vi "Trigger.vi"() -> ()   [LabVIEW 2014]
panel:
  in  "ICImagingControl":refnum<k7>(container)
  out "Picture Out":picture
  in  "Open Device Configuration (Monochrome  Images)":bool
  in  "Open Device Configuration (Color Images)":bool
  out "ReferenceTimeStart":dbl
  out "Image Age":dbl
  out "ReferenceTimeCurrent":dbl
  out "SampleStartTime":dbl
  in  "External Trigger":bool
  in  "Grab":bool
  in  "End Program":bool
  # "Open Device Configuration"
  # "Off"
  # "On"
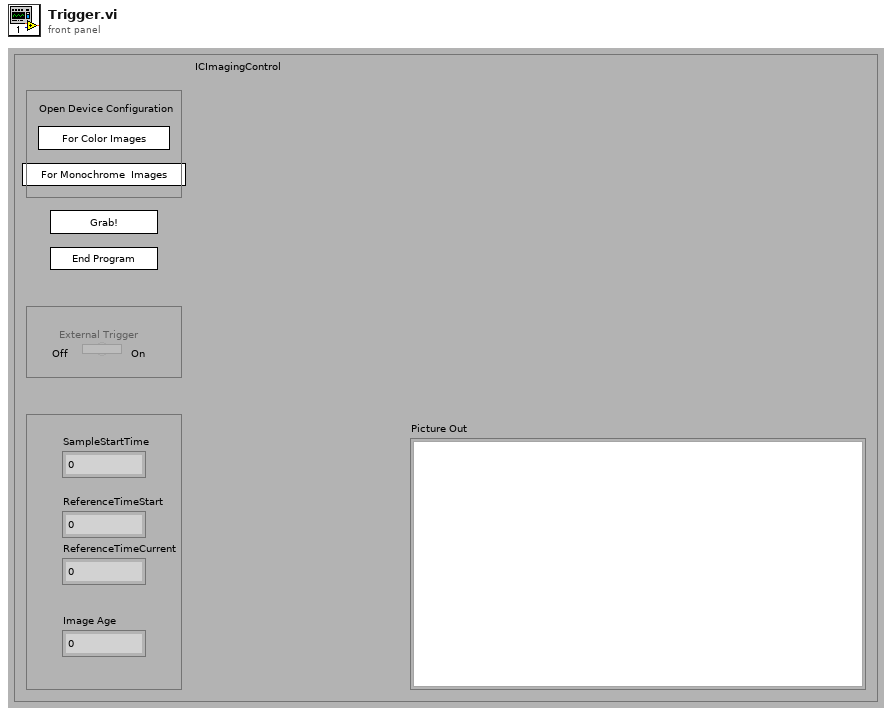
[diagram p1: front panel]
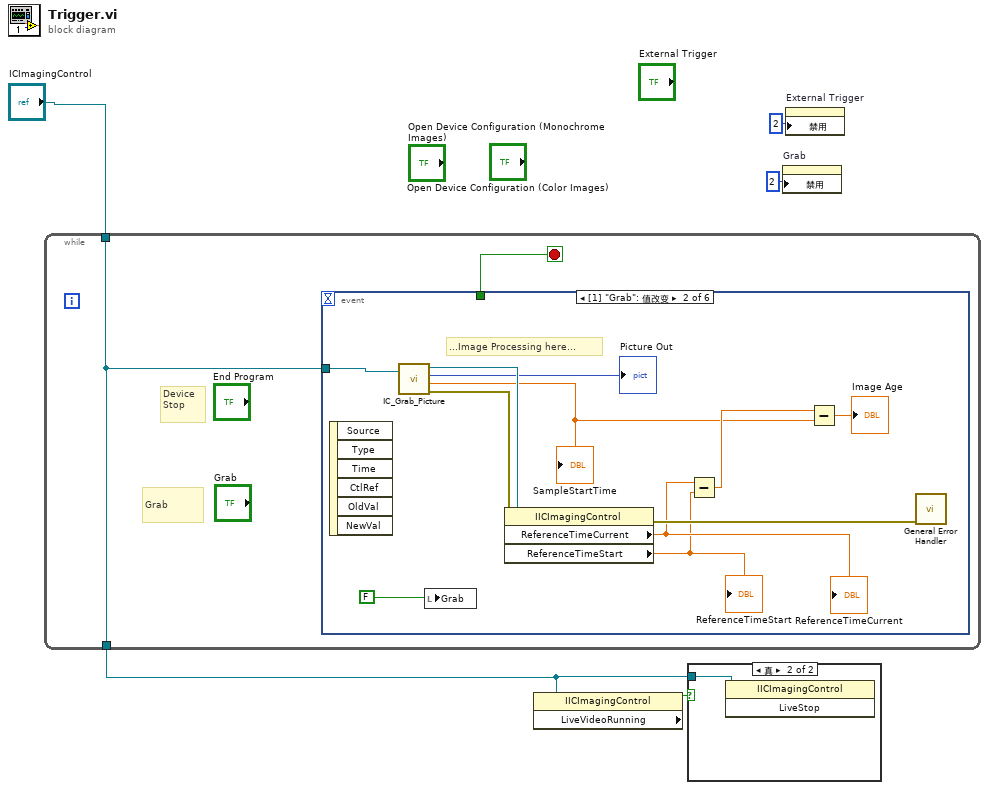
[diagram p0: block diagram]
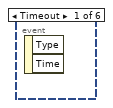
[diagram p3: hidden frame]
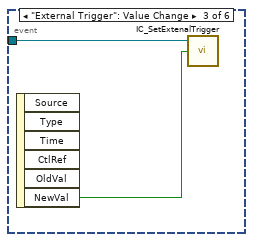
[diagram p4: hidden frame]
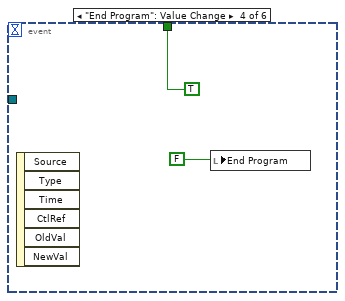
[diagram p5: hidden frame]
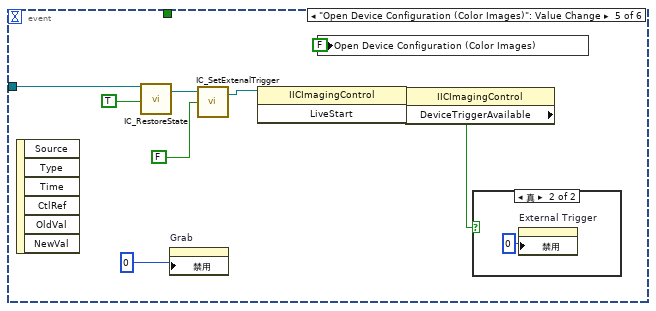
[diagram p6: hidden frame]
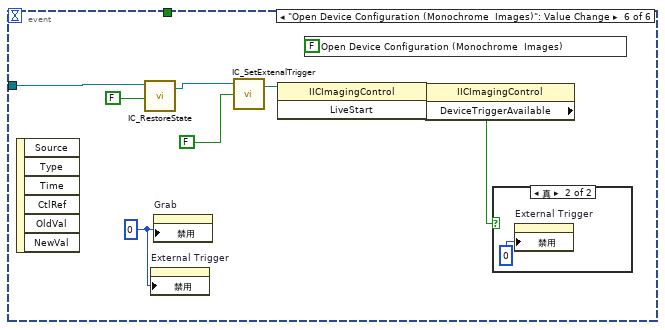
[diagram p8: hidden frame]
diagram:
  n1 = while {
    tunnel: "ICImagingControl" -> [w6]
    tunnel: [w6] -> w4
    stop <- w7 stop-if-true
    # "Device\nStop"
    # "Grab"
    n2 = event shown="[1] \"Grab\": 值改变" {
      selector: _ -> [_ _ _ _ _ _]
      dyn-events: _ -> [_ _ _ _ _ _]
      timeout: _ -> [_ _ _ _ _ _]
      tunnel: w6 -> [_ w17 w20 _ w31 w40]
      tunnel: [_ _ _ TRUE _ _] -> w7
      event Timeout {
        n3 = event-data() -> ()  [unwired: 1 in, 2 out]
      }
      event "Grab": Value Change {
        # "...Image Processing here..."
        n4 = event-data() -> ()  [unwired: 1 in, 6 out]
        n5 = call "IC_Grab_Picture.vi"("ICImagingControl In"=w17) -> ("ICImagingControl Out"=w16:refnum<k7>, "Picture Out"=→"Picture Out":picture, "SampleStartTime"=w11:dbl, "Error Out"=w13:errorcluster)  [unwired: 1 in]
        "SampleStartTime" <- w11
        n6 = local write "Grab"(FALSE) -> ()
        n7 = property class="IICImagingControl"(reference=w16, error in=w13) -> (error out=w14:errorcluster, "ReferenceTimeCurrent"=w10:dbl, "ReferenceTimeStart"=w9:dbl)  [unwired: 1 out]
        "ReferenceTimeCurrent" <- w10
        "ReferenceTimeStart" <- w9
        n8 = Subtract(x=w10, y=w9) -> (x-y=w12:dbl)
        n9 = Subtract(x=w12, y=w11) -> (x-y=→"Image Age":dbl)
        n10 = call <vilib>:"General Error Handler.vi"("error in (no error)"=w14) -> ()  [unwired: 10 in, 5 out]
      }
      event "External Trigger": Value Change {
        n11 = event-data() -> ("NewVal"=w19:bool)  [unwired: 1 in, 5 out]
        n12 = call <userlib>:"IC_SetExtenalTrigger.vi"("Trigger"=w19, "ICImagingControl In"=w20) -> ()  [unwired: 1 in, 2 out]
      }
      event "End Program": Value Change {
        n13 = event-data() -> ()  [unwired: 1 in, 6 out]
        n14 = local write "End Program"(FALSE) -> ()
      }
      event "Open Device Configuration (Color Images)": Value Change {
        n15 = event-data() -> ()  [unwired: 1 in, 6 out]
        n16 = call "IC_RestoreState.vi"("Color"=TRUE, "ICImagingControl"=w31) -> ("ICImagingControl Out"=w23:refnum<k7>)  [unwired: 2 in, 1 out]
        n17 = property on="Grab" class="Bool (严格)"("禁用"=0) -> ()  [unwired: 2 in, 2 out]
        n18 = call <userlib>:"IC_SetExtenalTrigger.vi"("Trigger"=FALSE, "ICImagingControl In"=w23) -> ("ICImagingControl Out"=w24:refnum<k7>)  [unwired: 1 in, 1 out]
        n19 = invoke class="IICImagingControl" method="LiveStart"(reference=w24) -> (reference out=w26:refnum<k7>)  [unwired: 2 in, 2 out]
        n20 = local write "Open Device Configuration (Color Images)"(FALSE ("Open Device Configuration (Color Images)")) -> ()
        n21 = property class="IICImagingControl"(reference=w26) -> ("DeviceTriggerAvailable"=w25:bool)  [unwired: 1 in, 2 out]
        n22 = case shown="真" w25 {
          frame False {
          }
          frame True {
            n23 = property on="External Trigger" class="Bool (严格)"("禁用"=u8 0 ("Disabled")) -> ()  [unwired: 2 in, 2 out]
          }
        }
      }
      event "Open Device Configuration (Monochrome  Images)": Value Change {
        w38 = 0
        n24 = event-data() -> ()  [unwired: 1 in, 6 out]
        n25 = call "IC_RestoreState.vi"("Color"=FALSE, "ICImagingControl"=w40) -> ("ICImagingControl Out"=w33:refnum<k7>)  [unwired: 2 in, 1 out]
        n26 = property on="External Trigger" class="Bool (严格)"("禁用"=w38) -> ()  [unwired: 2 in, 2 out]
        n27 = property on="Grab" class="Bool (严格)"("禁用"=w38) -> ()  [unwired: 2 in, 2 out]
        n28 = call <userlib>:"IC_SetExtenalTrigger.vi"("Trigger"=FALSE, "ICImagingControl In"=w33) -> ("ICImagingControl Out"=w36:refnum<k7>)  [unwired: 1 in, 1 out]
        n29 = invoke class="IICImagingControl" method="LiveStart"(reference=w36) -> (reference out=w35:refnum<k7>)  [unwired: 2 in, 2 out]
        n30 = local write "Open Device Configuration (Monochrome  Images)"(FALSE ("Open Device Configuration (Monochrome  Images)")) -> ()
        n31 = property class="IICImagingControl"(reference=w35) -> ("DeviceTriggerAvailable"=w34:bool)  [unwired: 1 in, 2 out]
        n32 = case shown="真" w34 {
          frame False {
          }
          frame True {
            n33 = property on="External Trigger" class="Bool (严格)"("禁用"=u8 0 ("Disabled")) -> ()  [unwired: 2 in, 2 out]
          }
        }
      }
    }
  }
  n34 = property class="IICImagingControl"(reference=w4) -> ("LiveVideoRunning"=w5:bool)  [unwired: 1 in, 2 out]
  n35 = case shown="真" w5 {
    tunnel: w4 -> [_ w43]
    frame False {
    }
    frame True {
      n36 = invoke class="IICImagingControl" method="LiveStop"(reference=w43) -> ()  [unwired: 2 in, 3 out]
    }
  }
  n37 = property on="Grab" class="Bool (严格)"("禁用"=u8 2 ("Disabled")) -> ()  [unwired: 2 in, 2 out]
  n38 = property on="External Trigger" class="Bool (严格)"("禁用"=u8 2 ("Disabled")) -> ()  [unwired: 2 in, 2 out]
